vi "Emit.vi"(8 "error in (no error)":errorcluster, 10 "response":T1, 11 "MultiResponder in":refnum<class "MultiResponder.lvclass">) -> (0 "error out":errorcluster, 3 "MultiResponder out":refnum<class "MultiResponder.lvclass">)   [LabVIEW 2013, in "MultiResponder.lvclass"]
doc: "Emit a response to the owning application"
uses:
  MultiResponder.lvclass
  response.ctl
  driver_status.ctl
  MultiResponder.lvclass/MultiResponder.ctl
  BaseResponder/BaseResponder.lvclass
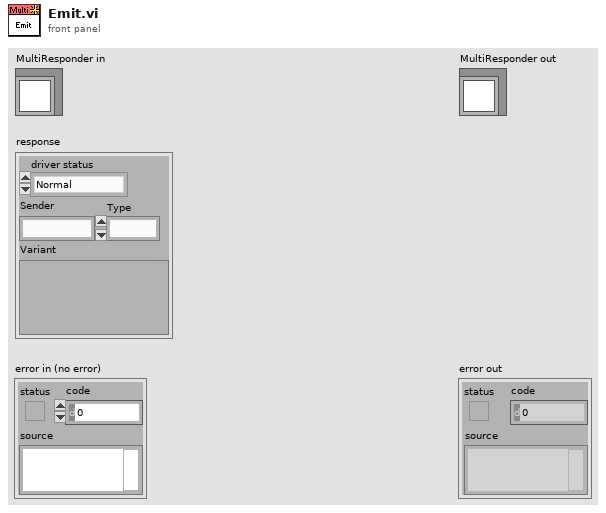
[diagram p1: front panel]
types:
  T1 = typedef "response.ctl" = cluster{"driver status":T2, "Sender":string, "Type":i32, "Variant":variant}
  T2 = typedef "driver_status.ctl" = enum16{"Normal", "Startup", "Connection lost", "Reconnected", "Timeout", "Idle", "Busy"}
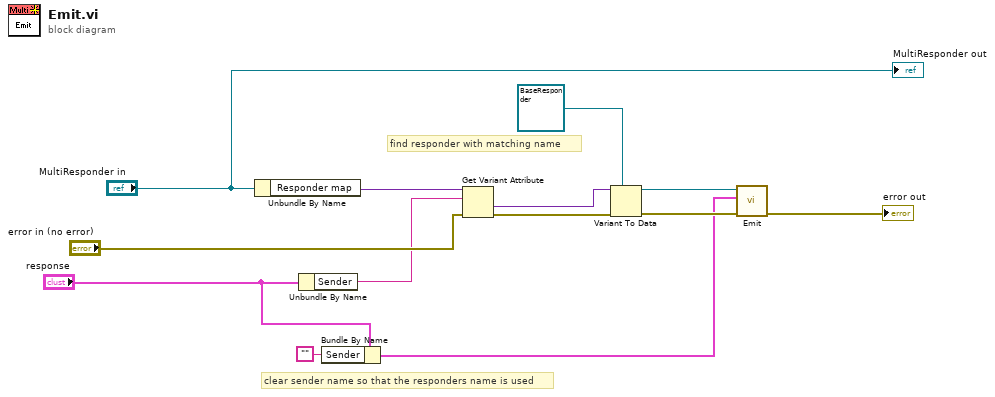
[diagram p0: block diagram]
diagram:
  # "clear sender name so that the responders name is used"
  # "find responder with matching name"
  n1 = Unbundle By Name("MultiResponder in") -> ("Responder map"=w3:variant)
  n2 = Unbundle By Name("response") -> ("Sender"=w4:string)
  n3 = Bundle By Name(cluster="response", "Sender"="") -> (w2:T1)
  n4 = Get Variant Attribute(Variant=w3, name=w4, error in="error in (no error)") -> (value=w7:variant, error out=w9:errorcluster)  [unwired: 1 in, 2 out]
  n5 = Variant To Data(error in=w9, type=refnum<class "BaseResponder.lvclass"> refnum ("BaseResponder.lvclass"), Variant=w7) -> (data=w8:refnum<class "BaseResponder.lvclass">, error out=w5:errorcluster)
  n6 = call-dynamic "Emit.vi"("error in (no error)"=w5, "response"=w2, "BaseResponder in"=w8) -> ("error out"=→"error out":errorcluster)  [unwired: 7 in, 1 out]
  "MultiResponder out" <- "MultiResponder in"
